vi "Teleop.vi"(10 "Match Info":T1={"Autonomous Elapsed Seconds"=0.0, "TeleOp Elapsed Seconds"=0.0, "Disabled Elapsed Seconds"=0.0, "Visited Autonomous"=FALSE, "Visited TeleOp"=FALSE, "Visited Disabled"=FALSE, "Autonomous Settings"={"Autonomous Style"=enum."Independent", "VI Refnum"=refnum}}, 11 "Call Context":T2) -> ()   [LabVIEW 2016]
doc: "This VI is called for each TeleOp packet received from the DS where the robot is not disabled. It is often used to read from the joysticks and update I/O or to update setpoints for timed control loops. It should complete and return within 20 milliseconds or it may miss DS packets."
uses:
  <vilib>/Rock Robotics/WPI/DriverStation/WPI_DriverStationDerivedRobotMode.ctl
  <vilib>/Rock Robotics/WPI/DriverStation/WPI_DriverStationMatch Info.ctl
  <vilib>/Rock Robotics/WPI/Solenoid/WPI_SolenoidValue.ctl
  <vilib>/Rock Robotics/Network Tables/NT Read Boolean.vi
  <vilib>/Rock Robotics/Network Tables/NT Read Number.vi
  Robot Global Data.vi
  Joystick Values.vi
  <vilib>/Rock Robotics/WPI/Solenoid/WPI_SolenoidSetEnum.vi
panel:
  in  "Max Shooter Speed":dbl=0.95
  out "Sample Slider 0":dbl(slide) scale=0.0..5.0
  out "Sample Boolean 1":bool
  out "Sample Boolean 0":bool
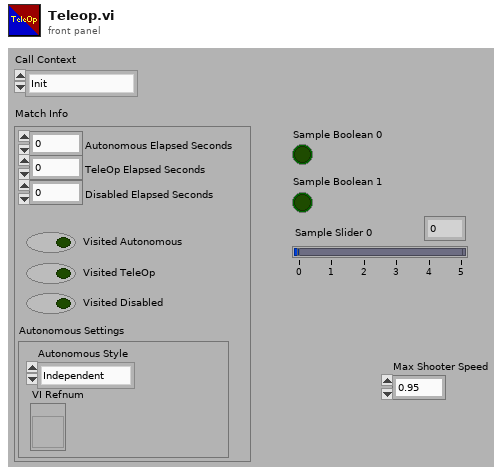
[diagram p1: front panel]
types:
  T1 = typedef "WPI_DriverStationMatch Info.ctl" = cluster{"Autonomous Elapsed Seconds":dbl, "TeleOp Elapsed Seconds":dbl, "Disabled Elapsed Seconds":dbl, "Visited Autonomous":bool, "Visited TeleOp":bool, "Visited Disabled":bool, "Autonomous Settings":cluster{"Autonomous Style":enum16{"Iterative", "Independent"}, "VI Refnum":refnum<vi>}}
  T2 = typedef "WPI_DriverStationDerivedRobotMode.ctl" = enum16{"Init", "Execute", "Stop"}
  T3 = typedef "WPI_SolenoidValue.ctl" = enum16{"Off", "On", "Forward", "Reverse"}
  T4 = typedef "WPI_MotorControlDeviceRef.ctl" = cluster{"DeviceStatus":errorcluster, "Type":T5, "PWM":cluster{"PWM Channel":T6, "DeadBand":T7}, "CAN":cluster{"Device Number":u8, "SetOutput VI Ref":variant, "GetOutput VI Ref":variant, "Enable VI Ref":variant, "Disable VI Ref":variant, "Data":variant}, "Invert":bool}
  T5 = typedef "WPI_MotorControlType.ctl" = enum16{"PWM", "CAN"}
  T6 = typedef "FPGA_DIOPWMChannel.ctl" = enum8{"PWM 0", "PWM 1", "PWM 2", "PWM 3", "PWM 4", "PWM 5", "PWM 6", "PWM 7", "PWM 8", "PWM 9", "PWM MXP 0", "PWM MXP 1", "PWM MXP 2", "PWM MXP 3", "PWM MXP 4", "PWM MXP 5", "PWM MXP 6", "PWM MXP 7", "PWM MXP 8", "PWM MXP 9", "Invalid"}
  T7 = typedef "WPI_PWMDeadband.ctl" = cluster{"Name":string, "maxPositivePwm":i32, "minPositivePwm":i32, "centerPwm":i32, "maxNegativePwm":i32, "minNegativePwm":i32, "angularRange":u16}
  T8 = typedef "WPI_SolenoidDevRef.ctl" = cluster{"DevStatus":errorcluster, "Pneumatics Control Module":u8, "Forward Solenoid Channel":T9, "Reverse Solenoid Channel":T9}
  T9 = typedef "WPI_SolenoidChannel.ctl" = enum8{"Solenoid 0", "Solenoid 1", "Solenoid 2", "Solenoid 3", "Solenoid 4", "Solenoid 5", "Solenoid 6", "Solenoid 7", "Invalid"}
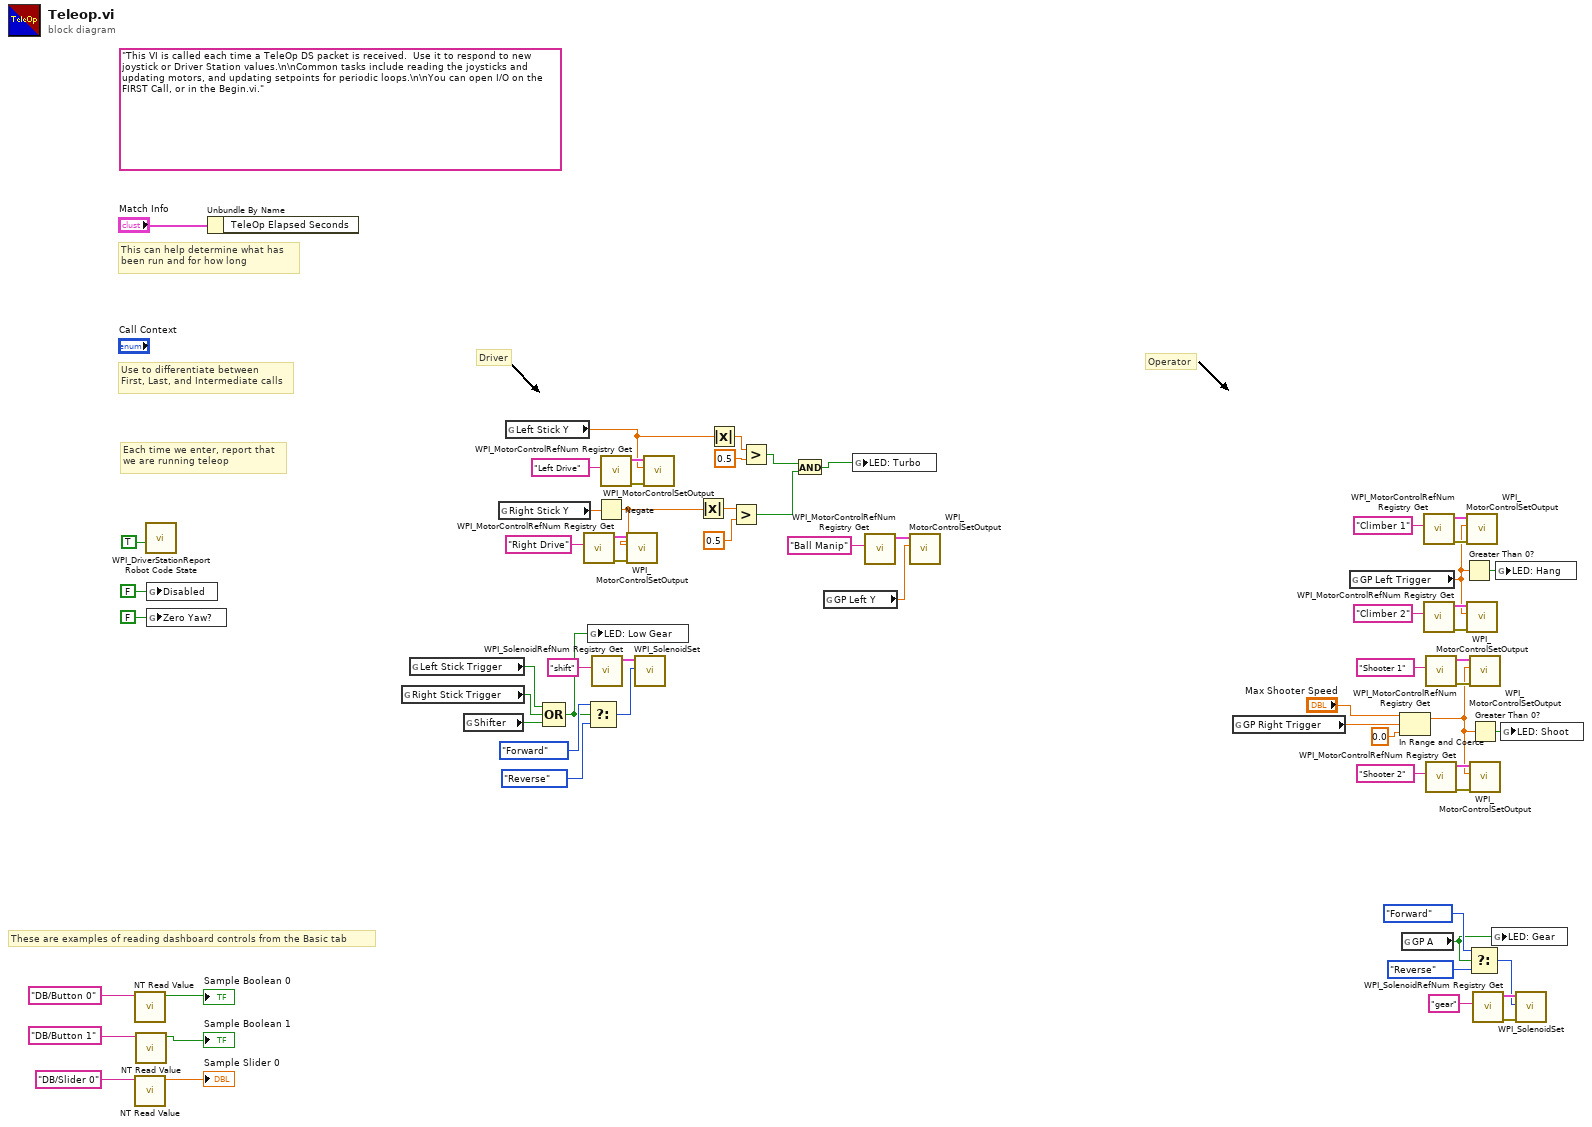
[diagram p0: block diagram]
diagram:
  (unwired) "This VI is called each time a TeleOp DS packet is received.  Use it to respond to new joystick or Driver Station values.\n\nCommon tasks include reading the joysticks and updating motors, and updating setpoints for periodic loops.\n\nYou can open I/O on the FIRST Call, or in the Begin.vi."
  # "Driver"
  # "Operator"
  # "These are examples of reading dashboard controls from the Basic tab"
  # "Each time we enter, report that\nwe are running teleop"
  # "Use to differentiate between\nFirst, Last, and Intermediate calls"
  # "This can help determine what has\nbeen run and for how long"
  n1 = call-poly <vilib>:"NT Read Value.vi"("Name"="DB/Button 0" ("refnum name")) -> ("Boolean"=→"Sample Boolean 0":bool)  [unwired: 9 in, 1 out]
  n2 = call-poly <vilib>:"NT Read Value.vi"("Name"="DB/Slider 0" ("refnum name")) -> ("Numeric"=→"Sample Slider 0":dbl)  [unwired: 9 in, 1 out]
  n3 = call-poly <vilib>:"NT Read Value.vi"("Name"="DB/Button 1" ("refnum name")) -> ("Boolean"=→"Sample Boolean 1":bool)  [unwired: 9 in, 1 out]
  n4 = call <vilib>:"WPI_DriverStationReport Robot Code State.vi"("TeleOp"=TRUE ("Autonomous")) -> ()  [unwired: 10 in, 1 out]
  n5 = global write "Robot Global Data.vi" "Disabled"(FALSE ("Disabled")) -> ()
  n6 = global write "Robot Global Data.vi" "Zero Yaw?"(FALSE) -> ()
  n7 = Unbundle By Name("Match Info") -> ()  [unwired: 1 out]
  n8 = global read "Joystick Values.vi" "Right Stick Trigger"() -> (w21:bool)
  n9 = global read "Joystick Values.vi" "Left Stick Trigger"() -> (w22:bool)
  n10 = global read "Joystick Values.vi" "Shifter"() -> (w20:bool)
  n11 = global read "Joystick Values.vi" "Right Stick Y"() -> (w23:dbl)
  n12 = global read "Joystick Values.vi" "Left Stick Y"() -> (w11:dbl)
  n13 = Compound Arithmetic op=OR(w22, w21, w20) -> (w15:bool)
  n14 = call <vilib>:"WPI_MotorControlRefNum Registry Get.vi"("refnum name"="Right Drive") -> ("error out"=w52:errorcluster, "MotorControlDevRef"=w53:T4)  [unwired: 9 in]
  n15 = global write "Robot Global Data.vi" "LED: Low Gear"(w15) -> ()
  n16 = Select(t=WPI_SolenoidValue."Forward" ("Value"), s=w15, f=WPI_SolenoidValue."Reverse" ("Value")) -> (s? t:f=w31:T3)
  n17 = call <vilib>:"WPI_SolenoidRefNum Registry Get.vi"("refnum name"="shift") -> ("SolenoidDevRef"=w34:T8)  [unwired: 9 in, 1 out]
  n18 = Negate(x=w23) -> (-x=w10:dbl)
  n19 = call <vilib>:"WPI_MotorControlRefNum Registry Get.vi"("refnum name"="Left Drive") -> ("error out"=w55:errorcluster, "MotorControlDevRef"=w56:T4)  [unwired: 9 in]
  n20 = call <vilib>:"WPI_MotorControlSetOutput.vi"("error in (no error)"=w52, "Output"=w10, "MotorControlDevRef"=w53) -> ()  [unwired: 6 in, 3 out]
  n21 = call-poly <vilib>:"WPI_SolenoidSet.vi"("Value"=w31, "SolenoidDevRef"=w34) -> ()  [unwired: 8 in, 2 out]
  n22 = call <vilib>:"WPI_MotorControlSetOutput.vi"("error in (no error)"=w55, "Output"=w11, "MotorControlDevRef"=w56) -> ()  [unwired: 6 in, 3 out]
  n23 = Absolute Value(x=w10) -> (abs(x)=w9:dbl)
  n24 = Absolute Value(x=w11) -> (abs(x)=w6:dbl)
  n25 = Greater?(x=w9, y=0.5) -> (0:w4:bool)
  n26 = Greater?(x=w6, y=0.5) -> (0:w5:bool)
  n27 = And(x=w5, y=w4) -> (x .and. y?=w3:bool)
  n28 = global read "Joystick Values.vi" "GP Left Y"() -> (w17:dbl)
  n29 = global write "Robot Global Data.vi" "LED: Turbo"(w3) -> ()
  n30 = call <vilib>:"WPI_MotorControlRefNum Registry Get.vi"("refnum name"="Ball Manip") -> ("MotorControlDevRef"=w19:T4)  [unwired: 9 in, 1 out]
  n31 = call <vilib>:"WPI_MotorControlSetOutput.vi"("Output"=w17, "MotorControlDevRef"=w19) -> ()  [unwired: 7 in, 3 out]
  n32 = global read "Joystick Values.vi" "GP Right Trigger"() -> (w47:dbl)
  n33 = global read "Joystick Values.vi" "GP Left Trigger"() -> (w1:dbl)
  n34 = In Range and Coerce(upper limit="Max Shooter Speed", x=w47, lower limit=0.0) -> (coerced(x)=w13:dbl)  [unwired: 1 out]
  n35 = global read "Joystick Values.vi" "GP A"() -> (w12:bool)
  n36 = call <vilib>:"WPI_MotorControlRefNum Registry Get.vi"("refnum name"="Climber 1") -> ("error out"=w43:errorcluster, "MotorControlDevRef"=w42:T4)  [unwired: 9 in]
  n37 = call <vilib>:"WPI_MotorControlRefNum Registry Get.vi"("refnum name"="Climber 2") -> ("error out"=w46:errorcluster, "MotorControlDevRef"=w45:T4)  [unwired: 9 in]
  n38 = call <vilib>:"WPI_MotorControlRefNum Registry Get.vi"("refnum name"="Shooter 1") -> ("error out"=w37:errorcluster, "MotorControlDevRef"=w36:T4)  [unwired: 9 in]
  n39 = call <vilib>:"WPI_MotorControlRefNum Registry Get.vi"("refnum name"="Shooter 2") -> ("error out"=w40:errorcluster, "MotorControlDevRef"=w39:T4)  [unwired: 9 in]
  n40 = Greater Than 0?(x=w1) -> (x > 0?=w2:bool)
  n41 = call <vilib>:"WPI_MotorControlSetOutput.vi"("error in (no error)"=w43, "Output"=w1, "MotorControlDevRef"=w42) -> ()  [unwired: 6 in, 3 out]
  n42 = call <vilib>:"WPI_MotorControlSetOutput.vi"("error in (no error)"=w46, "Output"=w1, "MotorControlDevRef"=w45) -> ()  [unwired: 6 in, 3 out]
  n43 = Select(t=WPI_SolenoidValue."Forward" ("Value"), s=w12, f=WPI_SolenoidValue."Reverse" ("Value")) -> (s? t:f=w26:T3)
  n44 = call <vilib>:"WPI_MotorControlSetOutput.vi"("error in (no error)"=w37, "Output"=w13, "MotorControlDevRef"=w36) -> ()  [unwired: 6 in, 3 out]
  n45 = Greater Than 0?(x=w13) -> (x > 0?=w14:bool)
  n46 = call <vilib>:"WPI_MotorControlSetOutput.vi"("error in (no error)"=w40, "Output"=w13, "MotorControlDevRef"=w39) -> ()  [unwired: 6 in, 3 out]
  n47 = call <vilib>:"WPI_SolenoidRefNum Registry Get.vi"("refnum name"="gear") -> ("error out"=w28:errorcluster, "SolenoidDevRef"=w29:T8)  [unwired: 9 in]
  n48 = global write "Robot Global Data.vi" "LED: Gear"(w12) -> ()
  n49 = global write "Robot Global Data.vi" "LED: Hang"(w2) -> ()
  n50 = global write "Robot Global Data.vi" "LED: Shoot"(w14) -> ()
  n51 = call-poly <vilib>:"WPI_SolenoidSet.vi"("error in (no error)"=w28, "Value"=w26, "SolenoidDevRef"=w29) -> ()  [unwired: 7 in, 2 out]
